vi "GlobalSetTemperaturCamera.vi"() -> ()   [LabVIEW 2011]
panel:
  in  "CameraTemperaturMinimumSet":dbl
  in  "CameraTemperaturMaximumSet":dbl
  in  "CameraTemperaturSet":dbl
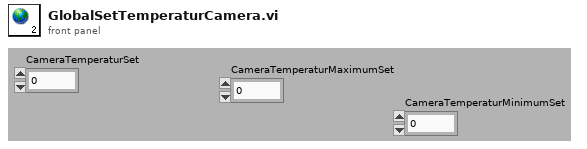
[diagram p1: front panel]
diagram:
